vi "AMI1700eth_init.vi"(8 "error in":errorcluster, 10 "port":u16, 11 "address":string) -> (0 "error out":errorcluster, 3 "conn_id":refnum<k5>, 4 "status":bool)   [LabVIEW 2019]
panel:
  out "ret3":string
  out "ret2":string
  out "ret1":string
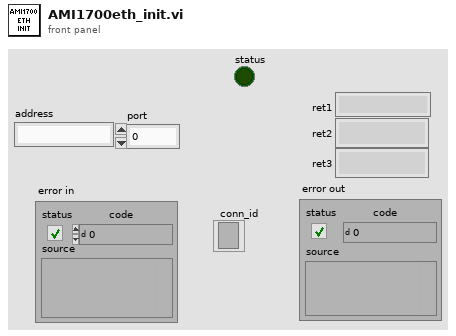
[diagram p1: front panel]
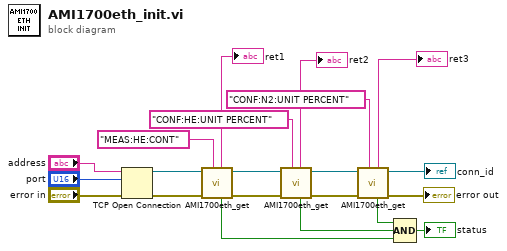
[diagram p0: block diagram]
diagram:
  n1 = TCP Open Connection(address="address", remote port or service name="port", error in (no error)="error in") -> (connection ID=w17:refnum<k5>, error out=w18:errorcluster)  [unwired: 2 in]
  n2 = call "AMI1700eth_get.vi"("command"="MEAS:HE:CONT", "error in"=w18, "conn_id_in"=w17) -> ("error out"=w13:errorcluster, "conn_id_out"=w14:refnum<k5>, "status"=w3:bool, "string"=→"ret1":string)  [unwired: 5 in]
  n3 = call "AMI1700eth_get.vi"("command"="CONF:HE:UNIT PERCENT", "error in"=w13, "conn_id_in"=w14) -> ("error out"=w11:errorcluster, "conn_id_out"=w12:refnum<k5>, "status"=w2:bool, "string"=→"ret2":string)  [unwired: 5 in]
  n4 = call "AMI1700eth_get.vi"("command"="CONF:N2:UNIT PERCENT", "error in"=w11, "conn_id_in"=w12) -> ("error out"=→"error out":errorcluster, "conn_id_out"=→"conn_id":refnum<k5>, "status"=w1:bool, "string"=→"ret3":string)  [unwired: 5 in]
  n5 = Compound Arithmetic op=AND(w1, w2, w3) -> (→"status":bool)
